vi "DropVI_MQTT Server.vi"() -> ()   [LabVIEW 2013]
uses:
  <vilib>/LabVIEW Open Source Project/MQTT Connection/MQTT_Connection/Connection/Connection.lvclass
  Server class/Server.lvclass/Server.ctl
  Server class/Server.lvclass
  <vilib>/LabVIEW Open Source Project/MQTT Connection/MQTT_Base/Base Class/MQTT_Base.lvclass
panel:
  out "error server":errorcluster
  out "NbConnections":u32
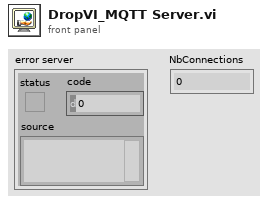
[diagram p1: front panel]
types:
  T1 = typedef "MQTT Server.lvlib/Server.lvclass/Public Events -- cluster.ctl" = cluster{"NbConnections":refnum<user-event>}
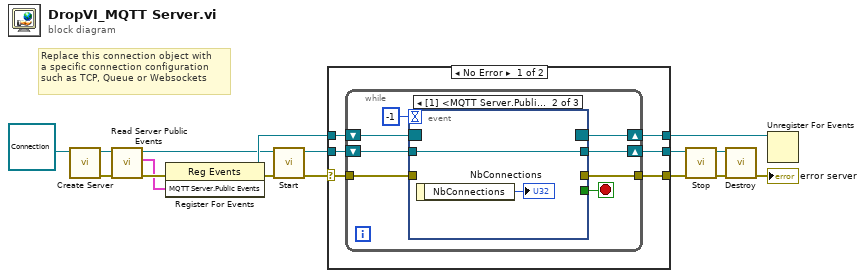
[diagram p0: block diagram]
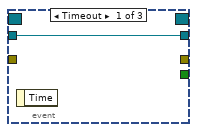
[diagram p2: hidden frame]
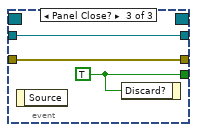
[diagram p3: hidden frame]
diagram:
  # "Replace this connection object with\na specific connection configuration\nsuch as TCP, Queue or Websockets"
  n1 = call "Create Server.vi"("Connection Configuration"=refnum<class "Connection.lvclass"> refnum) -> ("error out"=w15:errorcluster, "Server"=w16:refnum<class "Server.lvclass">)  [unwired: 9 in]
  n2 = call "Read Server Public Events.vi"("error in (no error)"=w15, "Server in"=w16) -> ("error out"=w14:errorcluster, "MQTT Server.Public Events"=w13:T1, "Server out"=w10:refnum<class "Server.lvclass">)  [unwired: 7 in]
  n3 = register-events(error in=w14, w13) -> (reference out=w12:refnum<event-registration>, error out=w8:errorcluster)  [unwired: 1 in]
  n4 = call <vilib>:"Start.vi"("error in (no error)"=w8, "MQTT_Base in"=w10) -> ("error out"=w7:errorcluster, "MQTT_Base out"=w9:refnum<class "Server.lvclass">)  [unwired: 7 in, 1 out]
  n5 = case shown="No Error" w7 {
    selector: w7 -> [w17 w37]
    tunnel: w9 -> [w22 w39]
    tunnel: [w21 w39] -> w3
    tunnel: w12 -> [w20 w38]
    tunnel: [w19 w38] -> w11
    tunnel: [w18 w37] -> w1
    frame No Error {
      n6 = while {
        shift-right: [w27] -> w21
        shift-left: w22 -> [w29]
        tunnel: [w24] -> w18
        tunnel: w17 -> [w23]
        shift-right: [w25] -> w19
        shift-left: w20 -> [w26]
        stop <- w28 stop-if-true
        n7 = event shown="[1] <MQTT Server.Public Events.NbConnections>: User Event" {
          selector: w26 -> [_ _ _]
          dyn-events: [_ _ _] -> w25
          timeout: -1 -> [_ _ _]
          tunnel: w29 -> [w31 w33 w36]
          tunnel: [_ _ w34] -> w28
          tunnel: [w31 w33 w36] -> w27
          tunnel: [_ _ w35] -> w24
          tunnel: w23 -> [_ _ w35]
          event Timeout {
            n8 = event-data() -> ()  [unwired: 1 in, 1 out]
          }
          event User Event {
            n9 = event-data() -> ("NbConnections"=→"NbConnections":u32)  [unwired: 1 in]
          }
          event Panel Close? {
            w34 = TRUE ("Discard?")
            n10 = event-data() -> ()  [unwired: 1 in, 1 out]
            n11 = event-data("Discard?"=w34) -> ()  [unwired: 1 in, 1 out]
          }
        }
      }
    }
    frame Error {
    }
  }
  n12 = call <vilib>:"Stop.vi"("error in (no error)"=w1, "MQTT_Base in"=w3) -> ("error out"=w2:errorcluster, "MQTT_Base out"=w4:refnum<class "Server.lvclass">)  [unwired: 7 in, 1 out]
  n13 = call <vilib>:"Destroy.vi"("error in (no error)"=w2, "MQTT_Base in"=w4) -> ("error out"=→"error server":errorcluster)  [unwired: 8 in, 1 out]
  n14 = Unregister For Events(event registration refnum=w11) -> ()  [unwired: 1 in, 1 out]
